vi "Add Image to Today's Page.vi"(8 "Error In (No Error)":errorcluster, 10 "Notebook Name":string="My notebook on One Drive", 11 "User Email":string="myemail") -> (0 "error out":errorcluster, 1 "body":string, 2 "headers":string, 3 "HTML with binary image data":string caption="Result")   [LabVIEW 2019, in "OneNote Library.lvlib"]
uses:
  OneNote Library.lvlib
  <vilib>/httpClient/MultipartData.ctl
  Useful OAuth VIs/globals.vi
  <vilib>/httpClient/LabVIEWHTTPClient.lvlib
  Useful OAuth VIs/Useful OAuth VIs.lvlib
panel:
  out "appended array":T1[](array[typedef])
  out "Page ID":string
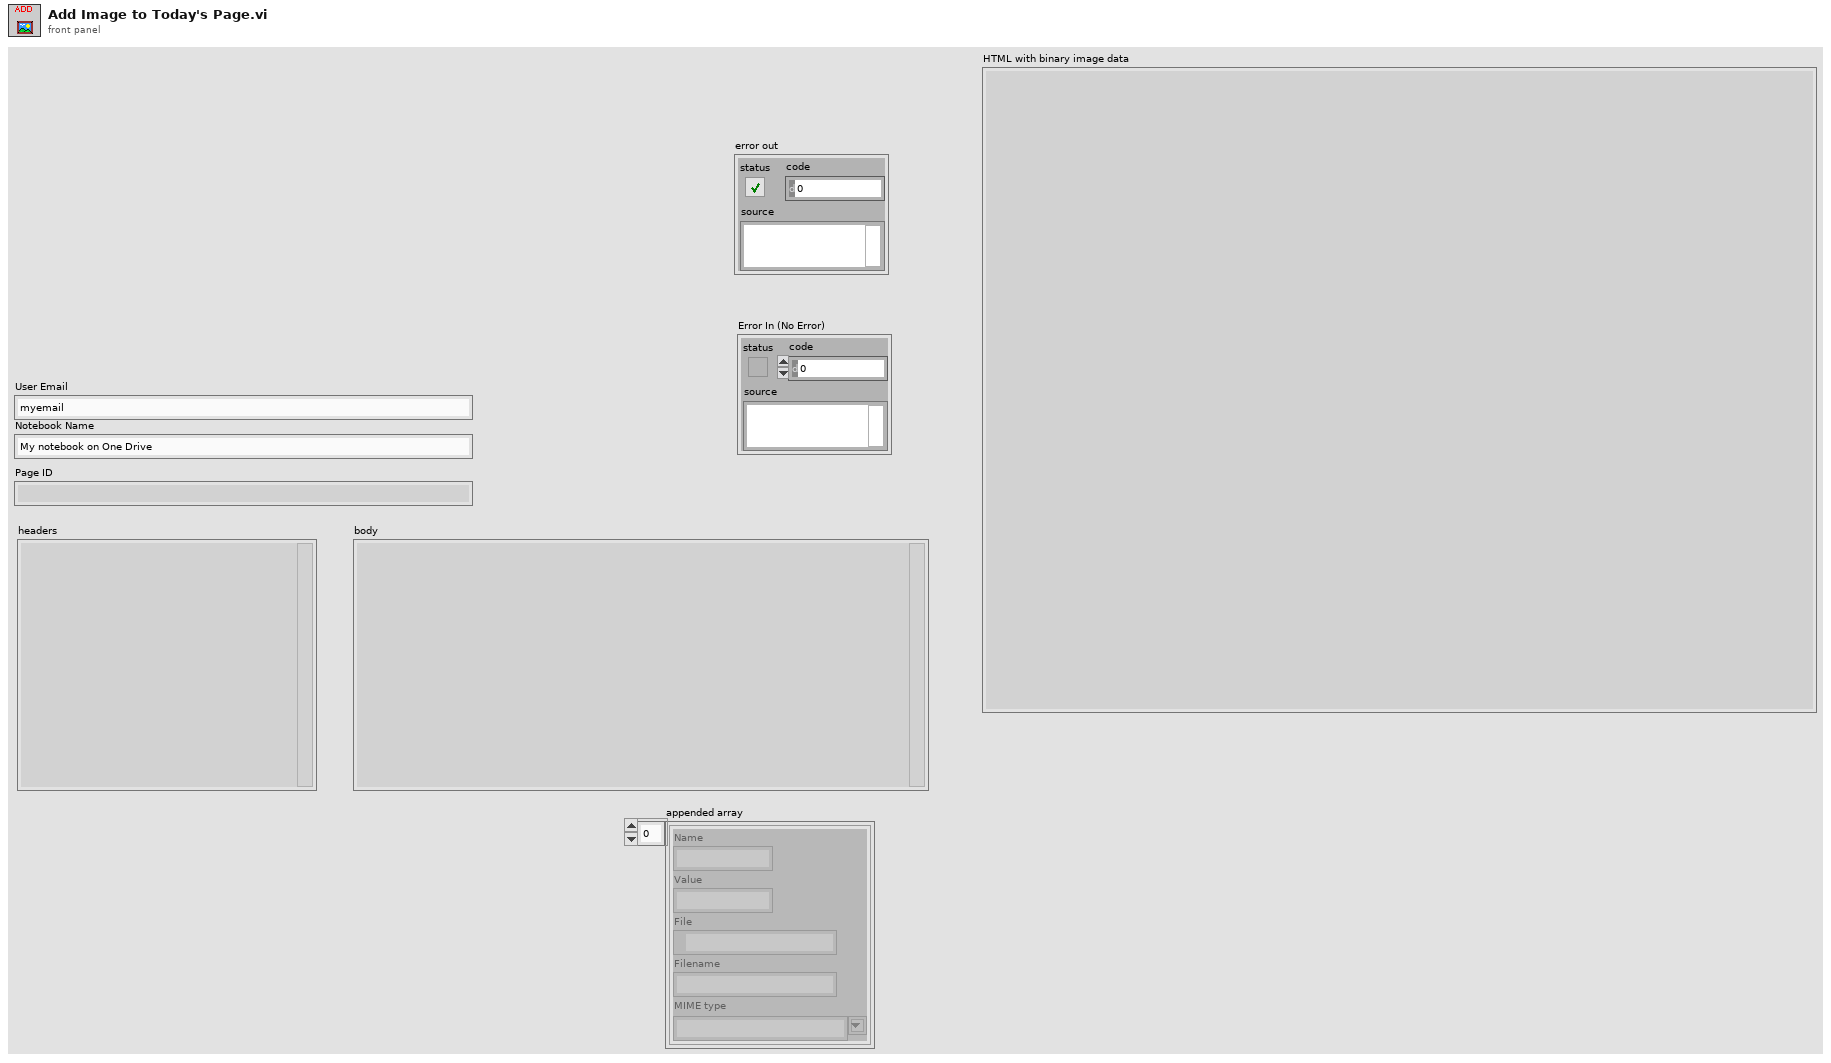
[diagram p1: front panel]
types:
  T1 = typedef "LabVIEWHTTPClient.lvlib/MultipartData.ctl" = cluster{"Name":string, "Value":string, "File":path, "Filename":string, "MIME type":string}
  T2 = typedef "LabVIEWHTTPClient.lvlib/ClientHandle.ctl" = refnum<k1>
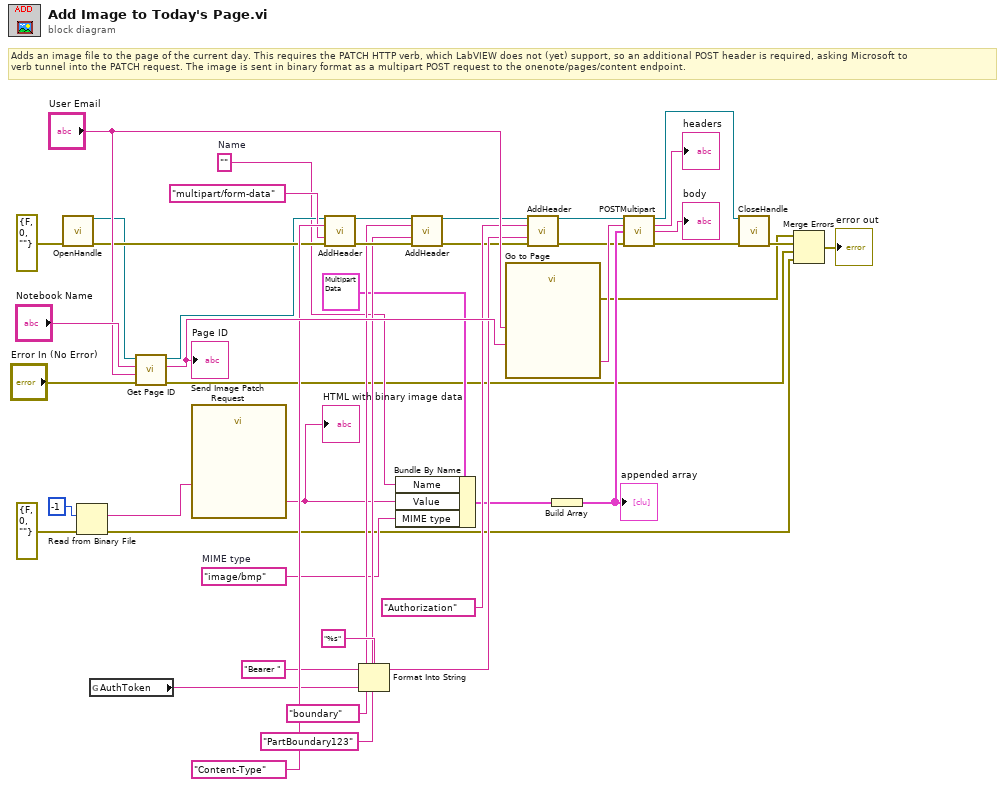
[diagram p0: block diagram]
diagram:
  w13 = "image/bmp"  # MIME type
  w14 = ""  # Name
  # "Adds an image file to the page of the current day. This requires the PATCH HTTP verb, which LabVIEW does not (yet) support, so an additional POST header is required, asking Microsoft to \nverb tunnel into the PATCH request. The image is sent in binary format as a multipart POST request to the onenote/pages/content endpoint."
  n1 = call <vilib>:"OpenHandle.vi"("error in (no error)"=errorcluster {"status"=FALSE, "code"=0, "source"=""}) -> ("client handle out"=w30:T2, "error out"=w36:errorcluster)  [unwired: 13 in]
  n2 = Read from Binary File(8:errorcluster {"status"=FALSE, "code"=0, "source"=""} ("error in"), 10:-1 ("count (1)")) -> (0:w4:errorcluster, 2:w1:string)  [unwired: 4 in, 2 out]
  n3 = global read "globals.vi" "AuthToken"() -> (w31:string)
  n4 = call "Get Page ID.vi"("Error In (No Error)"="Error In (No Error)", "User Email"="User Email", "Notebook Name"="Notebook Name", "client handle"=w30) -> ("error out"=w6:errorcluster, "Page ID"=w39:string, "client handle out"=w29:T2)  [unwired: 5 in]
  "Page ID" <- w39
  n5 = call "Send Image Patch Request"("Binary Image Data"=w1) -> ("Result"=w9:string)  [unwired: 13 in, 1 out]
  "HTML with binary image data" <- w9
  n6 = call <vilib>:"AddHeader.vi"("client handle"=w29, "header"="Content-Type", "value"="multipart/form-data", "error in (no error)"=w36) -> ("client handle out"=w23:T2, "error out"=w22:errorcluster)  [unwired: 10 in]
  n7 = Format Into String(format string="%s", initial string="Bearer ", w31) -> (resulting string=w32:string)  [unwired: 1 in, 1 out]
  n8 = Bundle By Name(cluster=T1 {"Name"="", "Value"="", "File"=path "", "Filename"="", "MIME type"="application/octet-stream"} ("Element"), "Name"=w14, "Value"=w9, "MIME type"=w13) -> (w12:T1)
  n9 = call <vilib>:"AddHeader.vi"("client handle"=w23, "header"="boundary", "value"="PartBoundary123", "error in (no error)"=w22) -> ("client handle out"=w21:T2, "error out"=w20:errorcluster)  [unwired: 10 in]
  n10 = call "Go to Page"("user"="User Email", "Page ID"=w39) -> ("Result"=w24:string, "error out"=w10:errorcluster)  [unwired: 12 in]
  n11 = call <vilib>:"AddHeader.vi"("client handle"=w21, "header"="Authorization", "value"=w32, "error in (no error)"=w20) -> ("client handle out"=w8:T2, "error out"=w7:errorcluster)  [unwired: 10 in]
  n12 = Build Array(w12) -> (w11:T1[])
  "appended array" <- w11
  n13 = call <vilib>:"POSTMultipart.vi"("client handle"=w8, "url"=w24, "data"=w11, "error in (no error)"=w7) -> ("client handle out"=w27:T2, "headers"=→"headers":string, "body"=→"body":string, "error out"=w28:errorcluster)  [unwired: 8 in]
  n14 = call <vilib>:"CloseHandle.vi"("client handle"=w27, "error in (no error)"=w28) -> ("error out"=w17:errorcluster)  [unwired: 13 in]
  n15 = Merge Errors(w10, w17, w6, w4) -> (→"error out":errorcluster)
